vi "Temperature Monitor.vi"() -> ()   [LabVIEW 2014]
doc: "本VI使用While循环和移位寄存器计算平均值。无需硬件。"
panel:
  in  "停止按钮":bool
  out "温度历史":dbl(graph)
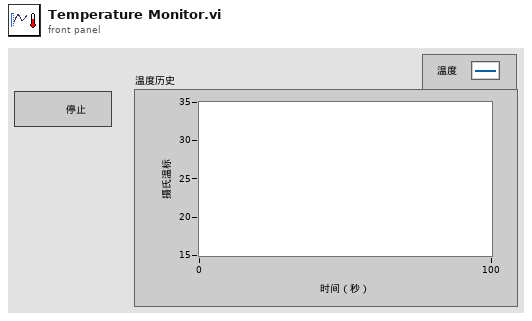
[diagram p1: front panel]
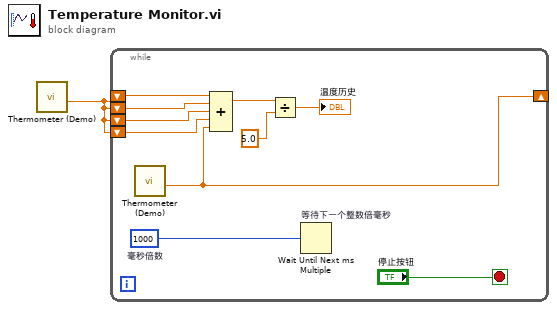
[diagram p0: block diagram]
diagram:
  n1 = call "Thermometer (Demo).vi"() -> ("温度值"=w1:dbl)  [unwired: 11 in]
  n2 = while {
    shift-right: [w6] -> _
    shift-left: w1 -> [w10]
    shift-left: w1 -> [w9]
    shift-left: w1 -> [w5]
    shift-left: w1 -> [w4]
    stop <- "停止按钮" stop-if-true
    w11 = u32 1000  # 毫秒倍数
    n3 = call "Thermometer (Demo).vi"() -> ("温度值"=w6:dbl)  [unwired: 11 in]
    n4 = Compound Arithmetic op=ADD(w10, w9, w5, w4, w6) -> (w8:dbl)
    n5 = Divide(x=w8, y=5.0) -> (x/y=→"温度历史":dbl)
    n6 = Wait Until Next ms Multiple "等待下一个整数倍毫秒"(millisecond multiple=w11) -> ()  [unwired: 1 out]
  }
